vi "String - Array Group By.vi"(11 "Array in":string[](array[string])) -> (3 "GROUP BY (Array in)":string[](array[string]))   [LabVIEW 2013]
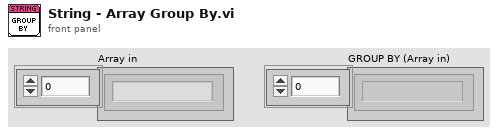
[diagram p1: front panel]
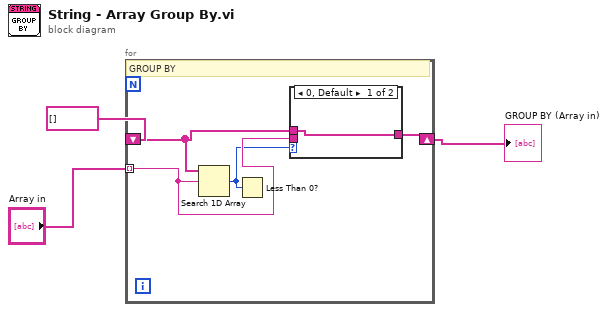
[diagram p0: block diagram]
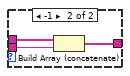
[diagram p2: hidden frame]
diagram:
  n1 = for {
    tunnel: "Array in" -> [w6] mode=indexing
    shift-right: [w5] -> w3
    shift-left: string[] [] -> [w7]
    # "GROUP BY"
    n2 = Search 1D Array(1D array=w7, element=w6) -> (index of element=w4:i32)  [unwired: 1 in]
    n3 = Less Than 0?(x=w4) -> ()  [unwired: 1 out]
    n4 = case shown="0, Default" w4 {
      tunnel: w7 -> [w8 w11]
      tunnel: w6 -> [_ w10]
      tunnel: [w8 w9] -> w5
      frame 0, Default {
      }
      frame -1 {
        n5 = Build Array (concatenate)(w11, w10) -> (w9:string[])
      }
    }
  }
  "GROUP BY (Array in)" <- w3
